vi "CreateRoomTable.vi"() -> ()   [LabVIEW 2015, in "DatabaseApi.lvlib"]
uses:
  DatabaseApi.lvlib
  TypeDef/Room/RoomTableDbTableName.ctl
  <vilib>/addons/database/Auxilliary.llb/DB Tools DataTypes.ctl
  TypeDef/Room/RoomTableColumnNames.ctl
  <vilib>/addons/database/Auxilliary.llb/DB Tools Column Info.ctl
  <vilib>/addons/database/Connection.llb/DB Tools Open Connec (Path).vi
  <vilib>/addons/database/NI_Database_API.lvlib
panel:
  in  "RoomTableName":T1="RoomTable"
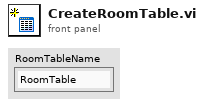
[diagram p1: front panel]
types:
  T1 = typedef "DatabaseApi.lvlib/RoomTableDbTableName.ctl" = string
  T2 = typedef "DatabaseApi.lvlib/RoomTableColumnNames.ctl" = string[]
  T3 = typedef "NI_Database_API.lvlib/DB Tools DataTypes.ctl" = enum16{"String", "Long (I32)", "Single (SGL)", "Double (DBL)", "Date/Time", "Binary"}
  T4 = typedef "NI_Database_API.lvlib/DB Tools Column Info.ctl" = cluster{"column name":string, "data type":T3, "size":i32, "allow null?":bool}
  T5 = typedef "NI_Database_API.lvlib/Conn ObjectReference.ctl" = refnum<k1>
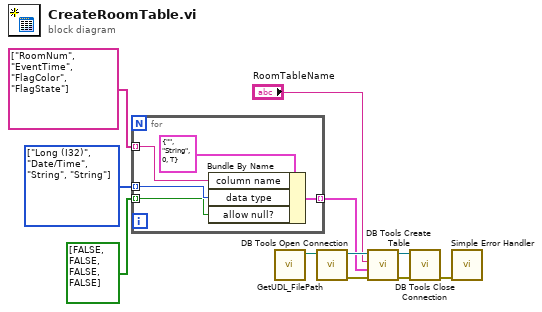
[diagram p0: block diagram]
diagram:
  w6 = T3[] [enum."Long (I32)", enum."Date/Time", enum."String", enum."String"] items=["String", "Long (I32)", "Single (SGL)", "Double (DBL)", "Date/Time", "Binary"] ("Array")
  n1 = for {
    tunnel: T2 ["RoomNum", "EventTime", "FlagColor", "FlagState"] ("Array") -> [w15] mode=indexing
    tunnel: w6 -> [w14] mode=indexing
    tunnel: bool[] [FALSE, FALSE, FALSE, FALSE] ("Array") -> [w13] mode=indexing
    tunnel: [w12] -> w4 mode=indexing
    n2 = Bundle By Name(cluster=T4 {"column name"="", "data type"=enum."String", "size"=0, "allow null?"=TRUE} ("column information"), "column name"=w15, "data type"=w14, "allow null?"=w13) -> (w12:T4)
  }
  n3 = call "GetUDL_FilePath.vi"() -> ("UDL file path"=w3:path)  [unwired: 11 in]
  n4 = call-poly <vilib>:"DB Tools Open Connection.vi"("connection information"=w3) -> ("error out"=w10:errorcluster, "connection reference"=w9:T5)  [unwired: 7 in]
  n5 = call <vilib>:"DB Tools Create Table.vi"("error in (no error)"=w10, "column information"=w4, "table"="RoomTableName", "connection reference"=w9) -> ("error out"=w8:errorcluster, "connection reference out"=w7:T5)  [unwired: 4 in]
  n6 = call <vilib>:"DB Tools Close Connection.vi"("error in (no error)"=w8, "connection reference"=w7) -> ("error out"=w11:errorcluster)  [unwired: 5 in]
  n7 = call <vilib>:"Simple Error Handler.vi"("error in (no error)"=w11) -> ()  [unwired: 4 in, 5 out]
